vi "Read THD Measurement.vi"(8 "error in (no error)":errorcluster, 10 "Analyzer (0: A0)":i32(ring) items=["A0", "A1"], 11 "VISA resource name":refnum<visa-resource-name>) -> (0 "error out":errorcluster, 1 "Measurement 2":dbl, 2 "Measurement 1":dbl, 3 "VISA resource name out":refnum<visa-resource-name>)   [LabVIEW 2014, in "Stanford Research SR1.lvlib"]
doc: "Reads the THD Digital Generator measurement."
uses:
  Stanford Research SR1.lvlib
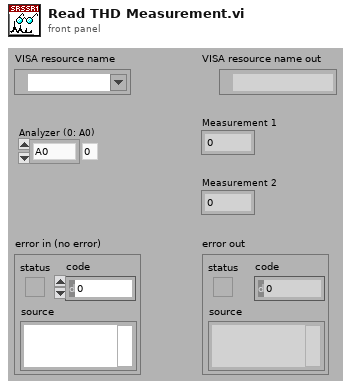
[diagram p1: front panel]
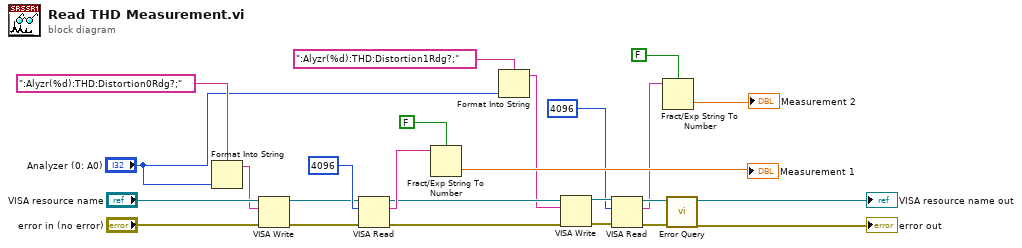
[diagram p0: block diagram]
diagram:
  n1 = Format Into String(format string=":Alyzr(%d):THD:Distortion0Rdg?;", "Analyzer (0: A0)") -> (resulting string=w17:string)  [unwired: 2 in, 1 out]
  n2 = VISA Write(VISA resource name="VISA resource name", write buffer=w17, error in (no error)="error in (no error)") -> (VISA resource name out=w22:refnum<visa-resource-name>, error out=w21:errorcluster)  [unwired: 1 out]
  n3 = VISA Read(VISA resource name=w22, byte count=u32 4096, error in (no error)=w21) -> (VISA resource name out=w12:refnum<visa-resource-name>, read buffer=w16:string, error out=w11:errorcluster)  [unwired: 1 out]
  n4 = Fract/Exp String To Number(use system decimal point (T)=FALSE, string=w16) -> (number=→"Measurement 1":dbl)  [unwired: 2 in, 1 out]
  n5 = Format Into String(format string=":Alyzr(%d):THD:Distortion1Rdg?;", "Analyzer (0: A0)") -> (resulting string=w10:string)  [unwired: 2 in, 1 out]
  n6 = VISA Write(VISA resource name=w12, write buffer=w10, error in (no error)=w11) -> (VISA resource name out=w9:refnum<visa-resource-name>, error out=w8:errorcluster)  [unwired: 1 out]
  n7 = VISA Read(VISA resource name=w9, byte count=u32 4096, error in (no error)=w8) -> (VISA resource name out=w7:refnum<visa-resource-name>, read buffer=w4:string, error out=w6:errorcluster)  [unwired: 1 out]
  n8 = Fract/Exp String To Number(use system decimal point (T)=FALSE, string=w4) -> (number=→"Measurement 2":dbl)  [unwired: 2 in, 1 out]
  n9 = call "Error Query.vi"("error in (no error)"=w6, "VISA resource name"=w7) -> ("error out"=→"error out":errorcluster, "VISA resource name out"=→"VISA resource name out":refnum<visa-resource-name>)  [unwired: 6 in, 2 out]
